vi "Request New Connection.vi"(8 "error in (no error)":errorcluster, 11 "PersistantConnectionHandler in":refnum<class "PersistantConnectionHandler.lvclass">) -> (0 "error out":errorcluster, 3 "PersistantConnectionHandler out":refnum<class "PersistantConnectionHandler.lvclass">)   [LabVIEW 2019, in "PersitantConnectionHandler.lvlib" / "PersistantConnectionHandler.lvclass"]
uses:
  <vilib>/gpm_packages/@cs/Network-interface/Source/PersistantConnectionHandler/PersistantConnectionHandler/PersistantConnectionHandler.lvclass
  C:/Program Files/National Instruments/LabVIEW 2019/vi.lib/ActorFramework/Actor/Actor.lvclass
  C:/Program Files/National Instruments/LabVIEW 2019/vi.lib/gpm_packages/@cs/Network-interface/Source/Logged Actor/LoggedActor.lvclass
  <vilib>/gpm_packages/@cs/event-logger/Source/Composed Log/Types/Log Level.ctl
  <vilib>/ActorFramework/Actor/Actor.lvclass/Actor.ctl
  <vilib>/ActorFramework/Message Enqueuer/Message Enqueuer.lvclass/Message Enqueuer.ctl
  <vilib>/gpm_packages/@cs/Network-interface/Source/Logged Actor/LoggedActor.lvclass/LoggedActor.ctl
  <vilib>/gpm_packages/@cs/event-logger/Source/Composed Log/LoggerReference/LoggerReference.lvclass/LoggerReference.ctl
  <vilib>/gpm_packages/@cs/Network-interface/Source/PersistantConnectionHandler/PersistantConnectionHandler/PersistantConnectionHandler.lvclass/PersistantConnectionHandler.ctl
  <vilib>/gpm_packages/@cs/Network-interface/Source/Connection Factory Session/ConnectionFactorySession/ConnectionFactorySession.lvclass/ConnectionFactorySession.ctl
  <vilib>/gpm_packages/@cs/Network-interface/Source/Connection Factory Session/Messages/Process Connection Msg/Process Connection Msg.lvclass/Process Connection Msg.ctl
  <vilib>/ActorFramework/Message Enqueuer/Init from Existing Queue.vi
  <vilib>/gpm_packages/@cs/event-logger/Source/Composed Log/LoggerReference/Log Event.vi
  <vilib>/gpm_packages/@cs/Network-interface/Source/Connection Factory Session/Messages/Process Connection Msg/Send New Connection.vi
  <vilib>/gpm_packages/@cs/event-logger/Source/Composed Log/LoggerReference/Log.vi
  <vilib>/gpm_packages/@cs/event-logger/Source/Composed Log/LoggerReference/Get Valid Event Time.vi
  <vilib>/ActorFramework/Message Enqueuer/Enqueue.vi
  <vilib>/gpm_packages/@cs/event-logger/Source/Composed Log/LoggerReference/Remove Stale Logs.vi
  <vilib>/gpm_packages/@cs/Network-interface/Source/PersistantConnectionHandler/New Connection Policy/New Connection Policy.lvclass
  C:/Program Files/National Instruments/LabVIEW 2019/vi.lib/gpm_packages/@cs/Network-interface/Source/Connection Factory Session/INewConnectionCallback/INewConnectionCallback.lvclass
  <vilib>/gpm_packages/@cs/Network-interface/Source/Connection Factory Session/Messages/Process Connection Msg/Process Connection Msg.lvclass
  C:/Program Files/National Instruments/LabVIEW 2019/vi.lib/ActorFramework/Message/Message.lvclass
  <vilib>/ActorFramework/Message Priority Queue/Priority Enqueue.vi
  <vilib>/ActorFramework/Message Enqueuer/Message Enqueuer.lvclass
  <vilib>/gpm_packages/@cs/Network-interface/Source/Connection Factory Session/ConnectionFactorySession/ConnectionFactorySession.lvclass
  <vilib>/ActorFramework/Actor/Actor.lvclass
  <vilib>/gpm_packages/@cs/Network-interface/Source/Logged Actor/LoggedActor.lvclass
  <vilib>/gpm_packages/@cs/event-logger/Source/Composed Log/Composed Log.lvlib
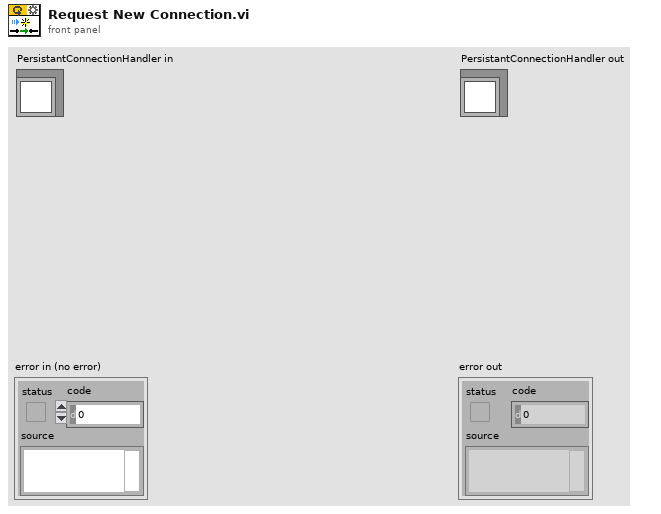
[diagram p1: front panel]
types:
  T1 = typedef "Composed Log.lvlib/Log Level.ctl" = enum16{"Debug", "Info", "Warning", "Error", "Critical"}
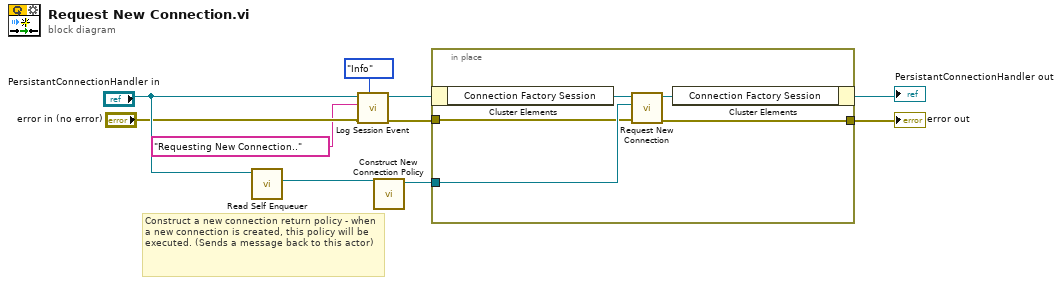
[diagram p0: block diagram]
diagram:
  # "Construct a new connection return policy - when a new connection is created, this policy will be executed. (Sends a message back to this actor)"
  n1 = call <vilib>:"Read Self Enqueuer.vi"("Actor"="PersistantConnectionHandler in") -> ("Self Enqueuer"=w6:refnum<class "Message Enqueuer.lvclass">)  [unwired: 10 in]
  n2 = call <vilib>:"Log Session Event.vi"("Event Level"=Log_Level."Info", "error in (no error)"="error in (no error)", "Event Data"="Requesting New Connection..", "SessionActor in"="PersistantConnectionHandler in") -> ("error out"=w3:errorcluster, "SessionActor out"=w5:refnum<class "PersistantConnectionHandler.lvclass">)  [unwired: 6 in]
  n3 = call <vilib>:"Construct New Connection Policy.vi"("Return Queue"=w6) -> ("New Connection Policy out"=w10:refnum<class "New Connection Policy.lvclass">)  [unwired: 10 in]
  n4 = in-place {
    in-place-border: w10 -> [w15]
    in-place-border: w3 -> [w12]
    in-place-border: [w11] -> w8
    n5 = in-place-cluster #1(w5) -> ("Connection Factory Session"=w14:refnum<data-value>)
    n6 = call <vilib>:"Request New Connection.vi"("error in (no error)"=w12, "New Connection Request"=w15, "Connection Factory Session In"=w14) -> ("error out"=w11:errorcluster, "Connection Factory Session Out"=w13:refnum<data-value>)  [unwired: 7 in]
    n7 = in-place-cluster #1("Connection Factory Session"=w13) -> (→"PersistantConnectionHandler out":refnum<class "PersistantConnectionHandler.lvclass">)
  }
  "error out" <- w8
